vi "MQTT_Subscribe.vi"(8 "error in (no error)":errorcluster, 9 "Message ID":u16=10 format="%x", 10 "Subscription Info Array":cluster{"Topic":string, "QoS":T1}[](array[cluster])=[{"Topic"="a/b", "QoS"=enum."At least once"}], 11 "connection ID":refnum<k5>) -> (0 "error out":errorcluster, 3 "connection ID out":refnum<k5>)   [LabVIEW 2025, in "MQTT_Functions.lvlib"]
doc: "This VI subscribes the client to a selected topic. The client now can read published messages for the topic. \n\n© 2015 - daq.io, LLC - Peter Adelhardt"
uses:
  MQTT_Functions.lvlib
  Controls/QoS.ctl
  Controls/MessageType.ctl
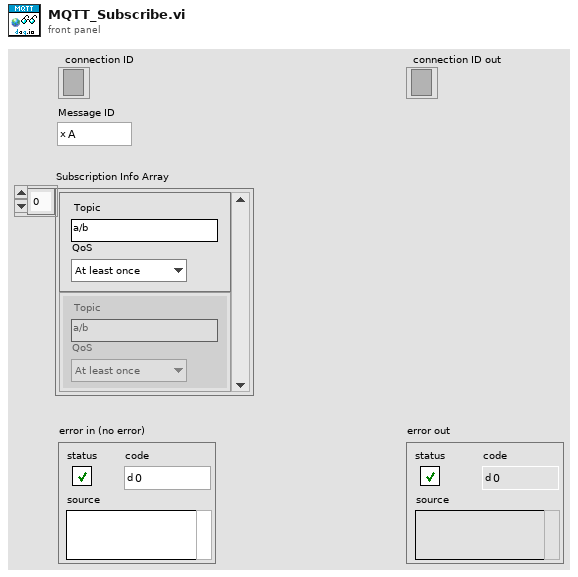
[diagram p1: front panel]
types:
  T1 = typedef "MQTT_Functions.lvlib/QoS.ctl" = enum8{"At most once", "At least once", "Exactly once", "Reserved"}
  T2 = typedef "MQTT_Functions.lvlib/MessageType.ctl" = enum32{"Reserved", "CONNECT", "CONNACK", "PUBLISH", "PUBACK", "PUBREC", "PUBREL", "PUBCOMP", "SUBSCRIBE", "SUBACK", "UNSUBSCRIBE", "UNSUBACK", "PINGREQ", "PINGRESP", "DISCONNECT", "Reserved2"}
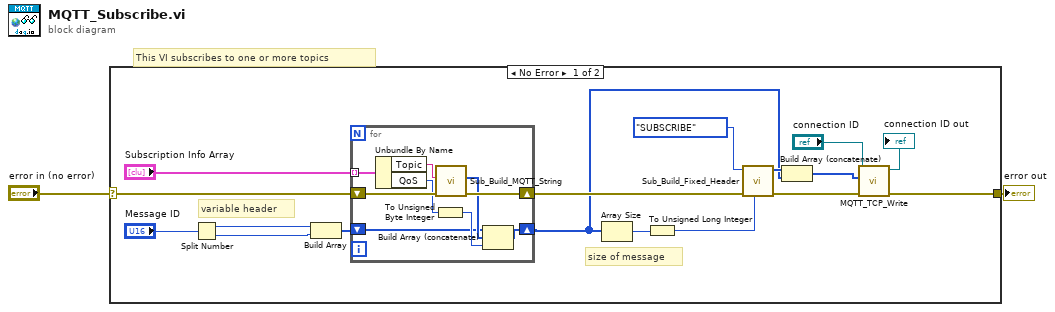
[diagram p0: block diagram]
diagram:
  # "This VI subscribes to one or more topics"
  n1 = case shown="No Error" "error in (no error)" {
    selector: "error in (no error)" -> [w12 w29]
    tunnel: [w6 w29] -> w1
    frame No Error {
      # "variable header"
      # "size of message"
      n2 = Split Number(x="Message ID") -> (hi(x)=w15:u8, lo(x)=w14:u8)
      n3 = Build Array(w15, w14) -> (w10:u8[])
      n4 = for {
        tunnel: "Subscription Info Array" -> [w28] mode=indexing
        shift-right: [w25] -> w9
        shift-left: w12 -> [w26]
        shift-right: [w21] -> w3
        shift-left: w10 -> [w20]
        n5 = Unbundle By Name(w28) -> ("Topic"=w27:string, "QoS"=w24:T1)
        n6 = To Unsigned Byte Integer(number=w24) -> (unsigned 8bit integer=w22:u8)
        n7 = call "Sub_Build_MQTT_String.vi"("error in (no error)"=w26, "String to be encoded"=w27) -> ("error out"=w25:errorcluster, "UTF8 Byte Array"=w23:u8[])  [unwired: 8 in]
        n8 = Build Array (concatenate)(w20, w23, w22) -> (w21:u8[])
      }
      n9 = Array Size(array=w3) -> (size(s)=w17:i32)
      n10 = To Unsigned Long Integer(number=w17) -> (unsigned 32bit integer=w18:u32)
      n11 = call "Sub_Build_Fixed_Header.vi"("Remaining Length"=w18, "error in (no error)"=w9, "MessageType"=MessageType."SUBSCRIBE") -> ("error out"=w7:errorcluster, "Fixed Header"=w16:u8[])  [unwired: 7 in]
      n12 = Build Array (concatenate)(w16, w3) -> (w8:u8[])
      n13 = call "MQTT_TCP_Write.vi"("error in (no error)"=w7, "data in"=w8, "connection ID"="connection ID") -> ("error out"=w6:errorcluster, "connection ID out"=→"connection ID out":refnum<k5>)  [unwired: 6 in, 1 out]
    }
    frame Error {
    }
  }
  "error out" <- w1
